vi "Auton_S1_Left_Scale_2Cube.vi"   [LabVIEW 2017]
uses:
  <vilib>/Rock Robotics/WPI/Utilities/WPI_GetSetVariantRefNum.vi
  Robot Global Data.vi
  <vilib>/Rock Robotics/WPI/RobotDrive/WPI_RobotDriveArcadeDrive_Standard(NoSaturation).vi
types:
  T1 = typedef "WPI_RobotDriveDevRef.ctl" = cluster{"DevStatus":errorcluster, "Motors[]":T2[], "Square Inputs":bool, "Max Output":dbl}
  T2 = typedef "WPI_MotorControlDeviceRef.ctl" = cluster{"DeviceStatus":errorcluster, "Type":T3, "PWM":cluster{"PWM Channel":T4, "DeadBand":T5}, "CAN":cluster{"Device Number":u8, "SetOutput VI Ref":variant, "GetOutput VI Ref":variant, "Enable VI Ref":variant, "Disable VI Ref":variant, "Data":variant}, "Invert":bool, "DIO PWM":cluster{"PWM \"Enable\" Channel":T4, "DIOChannel":T6, "PWM Rate":dbl}}
  T3 = typedef "WPI_MotorControlType.ctl" = enum16{"PWM", "CAN", "DIO PWM"}
  T4 = typedef "FPGA_DIOPWMChannel.ctl" = enum8{"PWM 0", "PWM 1", "PWM 2", "PWM 3", "PWM 4", "PWM 5", "PWM 6", "PWM 7", "PWM 8", "PWM 9", "PWM MXP 0", "PWM MXP 1", "PWM MXP 2", "PWM MXP 3", "PWM MXP 4", "PWM MXP 5", "PWM MXP 6", "PWM MXP 7", "PWM MXP 8", "PWM MXP 9", "Invalid"}
  T5 = typedef "WPI_PWMDeadband.ctl" = cluster{"Name":string, "maxPositivePwm":i32, "minPositivePwm":i32, "centerPwm":i32, "maxNegativePwm":i32, "minNegativePwm":i32, "angularRange":u16}
  T6 = typedef "FPGA_DIOChannel.ctl" = enum8{"DIO 0", "DIO 1", "DIO 2", "DIO 3", "DIO 4", "DIO 5", "DIO 6", "DIO 7", "DIO 8", "DIO 9", "DIO MXP 0", "DIO MXP 1", "DIO MXP 2", "DIO MXP 3", "DIO MXP 4", "DIO MXP 5", "DIO MXP 6", "DIO MXP 7", "DIO MXP 8", "DIO MXP 9", "DIO MXP 10", "DIO MXP 11", "DIO MXP 12", "DIO MXP 13", "DIO MXP 14", "DIO MXP 15", "SPI Port CS1", "SPI Port CS2", "SPI Port CS3", "SPI Port MISO", "SPI Port MOSI", "Invalid"}
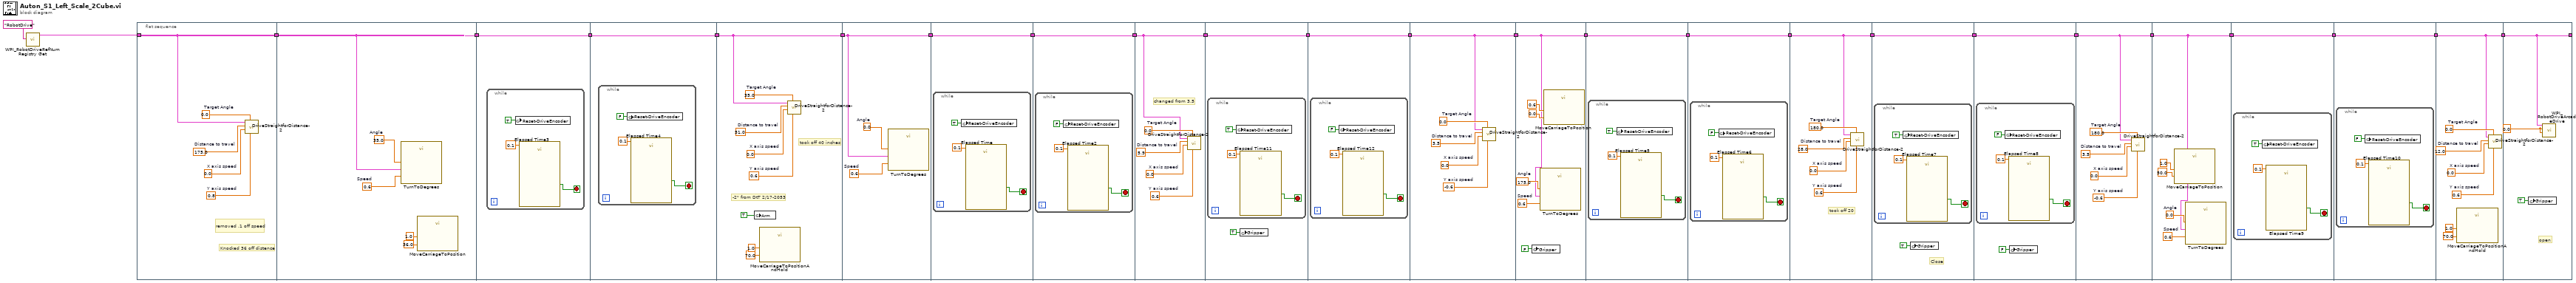
[diagram p0: block diagram]
diagram:
  n1 = call <vilib>:"WPI_RobotDriveRefNum Registry Get.vi"("refnum name"="RobotDrive") -> ("RobotDriveDevRef"=w22:T1)  [unwired: 9 in, 1 out]
  n2 = flat-sequence {
    tunnel: [w30] -> w1
    tunnel: w22 -> [w30]
    tunnel: [w34] -> w25
    tunnel: w1 -> [w34]
    tunnel: w25 -> [w36]
    tunnel: [w36] -> w24
    tunnel: [w40] -> w21
    tunnel: w24 -> [w40]
    tunnel: w21 -> [w47]
    tunnel: [w47] -> w7
    tunnel: w7 -> [w52]
    tunnel: [w52] -> w6
    tunnel: w6 -> [w55]
    tunnel: [w55] -> w20
    tunnel: w20 -> [w59]
    tunnel: [w59] -> w19
    tunnel: w19 -> [w63]
    tunnel: [w63] -> w5
    tunnel: w5 -> [w69]
    tunnel: [w69] -> w3
    tunnel: w3 -> [w73]
    tunnel: [w73] -> w2
    tunnel: w2 -> [w77]
    tunnel: [w77] -> w4
    tunnel: w4 -> [w83]
    tunnel: [w83] -> w18
    tunnel: w18 -> [w88]
    tunnel: [w88] -> w17
    tunnel: w17 -> [w92]
    tunnel: [w92] -> w16
    tunnel: w16 -> [w96]
    tunnel: [w96] -> w15
    tunnel: w15 -> [w102]
    tunnel: [w102] -> w14
    tunnel: w14 -> [w107]
    tunnel: [w107] -> w13
    tunnel: w13 -> [w111]
    tunnel: [w111] -> w12
    tunnel: w12 -> [w118]
    tunnel: [w118] -> w11
    tunnel: w11 -> [w121]
    tunnel: [w121] -> w10
    tunnel: w10 -> [w125]
    tunnel: [w125] -> w9
    tunnel: w9 -> [w131]
    tunnel: [w131] -> w8
    tunnel: [w137] -> _
    tunnel: w8 -> [w137]
    frame #0 {
      w26 = 0.0  # Target Angle
      w27 = 0.8  # Y axis speed
      w28 = 0.0  # X axis speed
      w29 = 175.0  # Distance to travel
      # "removed .1 off speed"
      # "Knocked 36 off distence"
      n3 = call "DriveStraightforDistance-2.vi"("Y axis speed"=w27, "Target Angle"=w26, "X axis speed"=w28, "Distance to travel"=w29, "RobotDriveDevRef"=w30) -> ()  [unwired: 7 in]
    }
    frame #1 {
      w33 = 35.0  # Angle
      w35 = 0.6  # Speed
      n4 = call "TurnToDegrees.vi"("Speed"=w35, "RobotDriveDevRef"=w34, "Angle"=w33) -> ()  [unwired: 9 in]
      n5 = call "MoveCarriageToPosition.vi"("Lift Speed"=1.0, "Target Height"=36.0) -> ()  [unwired: 10 in]
    }
    frame #2 {
      n6 = while {
        stop <- w39 stop-if-true
        n7 = global write "Robot Global Data.vi" "Reset-DriveEncoder"(TRUE ("Reset-DriveEncoder")) -> ()
        n8 = call "Elapsed Time3"("Time Target (s)"=0.1) -> ("Time has Elapsed"=w39:bool)  [unwired: 11 in, 7 out]
      }
    }
    frame #3 {
      n9 = while {
        stop <- w43 stop-if-true
        n10 = global write "Robot Global Data.vi" "Reset-DriveEncoder"(FALSE ("Reset-DriveEncoder")) -> ()
        n11 = call "Elapsed Time4"("Time Target (s)"=0.1) -> ("Time has Elapsed"=w43:bool)  [unwired: 11 in, 7 out]
      }
    }
    frame #4 {
      w48 = 35.0  # Target Angle
      w49 = 0.6  # Y axis speed
      w50 = 0.0  # X axis speed
      w51 = 51.0  # Distance to travel
      # "took off 40 inches"
      # "-2\" from DtT 2/17-2053"
      n12 = global write "Robot Global Data.vi" "Arm"(TRUE ("Gripper")) -> ()
      n13 = call "MoveCarriageToPositionAndHold.vi"("Lift Speed"=1.0, "Target Height"=70.0) -> ()  [unwired: 10 in]
      n14 = call "DriveStraightforDistance-2.vi"("Y axis speed"=w49, "Target Angle"=w48, "X axis speed"=w50, "Distance to travel"=w51, "RobotDriveDevRef"=w47) -> ()  [unwired: 7 in]
    }
    frame #5 {
      w53 = 0.0  # Angle
      w54 = 0.6  # Speed
      n15 = call "TurnToDegrees.vi"("Speed"=w54, "RobotDriveDevRef"=w52, "Angle"=w53) -> ()  [unwired: 9 in]
    }
    frame #6 {
      n16 = while {
        stop <- w58 stop-if-true
        n17 = global write "Robot Global Data.vi" "Reset-DriveEncoder"(TRUE ("Reset-DriveEncoder")) -> ()
        n18 = call "Elapsed Time"("Time Target (s)"=0.1) -> ("Time has Elapsed"=w58:bool)  [unwired: 11 in, 7 out]
      }
    }
    frame #7 {
      n19 = while {
        stop <- w62 stop-if-true
        n20 = global write "Robot Global Data.vi" "Reset-DriveEncoder"(FALSE ("Reset-DriveEncoder")) -> ()
        n21 = call "Elapsed Time2"("Time Target (s)"=0.1) -> ("Time has Elapsed"=w62:bool)  [unwired: 11 in, 7 out]
      }
    }
    frame #8 {
      w64 = 0.0  # Target Angle
      w65 = 0.6  # Y axis speed
      w66 = 0.0  # X axis speed
      w67 = 5.9  # Distance to travel
      # "changed from 3.5"
      n22 = call "DriveStraightforDistance-2.vi"("Y axis speed"=w65, "Target Angle"=w64, "X axis speed"=w66, "Distance to travel"=w67, "RobotDriveDevRef"=w63) -> ()  [unwired: 7 in]
    }
    frame #9 {
      n23 = while {
        stop <- w72 stop-if-true
        n24 = global write "Robot Global Data.vi" "Reset-DriveEncoder"(TRUE ("Reset-DriveEncoder")) -> ()
        n25 = call "Elapsed Time11"("Time Target (s)"=0.1) -> ("Time has Elapsed"=w72:bool)  [unwired: 11 in, 7 out]
      }
      n26 = global write "Robot Global Data.vi" "Gripper"(TRUE ("Gripper")) -> ()
    }
    frame #10 {
      n27 = while {
        stop <- w76 stop-if-true
        n28 = global write "Robot Global Data.vi" "Reset-DriveEncoder"(FALSE ("Reset-DriveEncoder")) -> ()
        n29 = call "Elapsed Time12"("Time Target (s)"=0.1) -> ("Time has Elapsed"=w76:bool)  [unwired: 11 in, 7 out]
      }
    }
    frame #11 {
      w78 = 0.0  # Target Angle
      w79 = -0.6  # Y axis speed
      w80 = 0.0  # X axis speed
      w81 = 3.5  # Distance to travel
      n30 = call "DriveStraightforDistance-2.vi"("Y axis speed"=w79, "Target Angle"=w78, "X axis speed"=w80, "Distance to travel"=w81, "RobotDriveDevRef"=w77) -> ()  [unwired: 7 in]
    }
    frame #12 {
      w84 = 175.0  # Angle
      w85 = 0.6  # Speed
      n31 = global write "Robot Global Data.vi" "Gripper"(FALSE ("Gripper")) -> ()
      n32 = call "TurnToDegrees.vi"("Speed"=w85, "RobotDriveDevRef"=w83, "Angle"=w84) -> ()  [unwired: 9 in]
      n33 = call "MoveCarriageToPosition.vi"("Lift Speed"=0.6, "Target Height"=0.0) -> ()  [unwired: 10 in]
    }
    frame #13 {
      n34 = while {
        stop <- w91 stop-if-true
        n35 = global write "Robot Global Data.vi" "Reset-DriveEncoder"(TRUE ("Reset-DriveEncoder")) -> ()
        n36 = call "Elapsed Time5"("Time Target (s)"=0.1) -> ("Time has Elapsed"=w91:bool)  [unwired: 11 in, 7 out]
      }
    }
    frame #14 {
      n37 = while {
        stop <- w95 stop-if-true
        n38 = global write "Robot Global Data.vi" "Reset-DriveEncoder"(FALSE ("Reset-DriveEncoder")) -> ()
        n39 = call "Elapsed Time6"("Time Target (s)"=0.1) -> ("Time has Elapsed"=w95:bool)  [unwired: 11 in, 7 out]
      }
    }
    frame #15 {
      w97 = 180.0  # Target Angle
      w98 = 0.6  # Y axis speed
      w99 = 0.0  # X axis speed
      w100 = 28.0  # Distance to travel
      # "took off 20"
      n40 = call "DriveStraightforDistance-2.vi"("Y axis speed"=w98, "Target Angle"=w97, "X axis speed"=w99, "Distance to travel"=w100, "RobotDriveDevRef"=w96) -> ()  [unwired: 7 in]
    }
    frame #16 {
      # "Close"
      n41 = while {
        stop <- w105 stop-if-true
        n42 = global write "Robot Global Data.vi" "Reset-DriveEncoder"(TRUE ("Reset-DriveEncoder")) -> ()
        n43 = call "Elapsed Time7"("Time Target (s)"=0.1) -> ("Time has Elapsed"=w105:bool)  [unwired: 11 in, 7 out]
      }
      n44 = global write "Robot Global Data.vi" "Gripper"(TRUE ("Gripper")) -> ()
    }
    frame #17 {
      n45 = while {
        stop <- w110 stop-if-true
        n46 = global write "Robot Global Data.vi" "Reset-DriveEncoder"(FALSE ("Reset-DriveEncoder")) -> ()
        n47 = call "Elapsed Time8"("Time Target (s)"=0.1) -> ("Time has Elapsed"=w110:bool)  [unwired: 11 in, 7 out]
      }
      n48 = global write "Robot Global Data.vi" "Gripper"(FALSE ("Gripper")) -> ()
    }
    frame #18 {
      w112 = 180.0  # Target Angle
      w113 = -0.6  # Y axis speed
      w114 = 0.0  # X axis speed
      w115 = 3.5  # Distance to travel
      n49 = call "DriveStraightforDistance-2.vi"("Y axis speed"=w113, "Target Angle"=w112, "X axis speed"=w114, "Distance to travel"=w115, "RobotDriveDevRef"=w111) -> ()  [unwired: 7 in]
    }
    frame #19 {
      w119 = 0.0  # Angle
      w120 = 0.6  # Speed
      n50 = call "MoveCarriageToPosition.vi"("Lift Speed"=1.0, "Target Height"=50.0) -> ()  [unwired: 10 in]
      n51 = call "TurnToDegrees.vi"("Speed"=w120, "RobotDriveDevRef"=w118, "Angle"=w119) -> ()  [unwired: 9 in]
    }
    frame #20 {
      n52 = while {
        stop <- w124 stop-if-true
        n53 = global write "Robot Global Data.vi" "Reset-DriveEncoder"(TRUE ("Reset-DriveEncoder")) -> ()
        n54 = call "Elapsed Time9"("Time Target (s)"=0.1) -> ("Time has Elapsed"=w124:bool)  [unwired: 11 in, 7 out]
      }
    }
    frame #21 {
      n55 = while {
        stop <- w128 stop-if-true
        n56 = global write "Robot Global Data.vi" "Reset-DriveEncoder"(FALSE ("Reset-DriveEncoder")) -> ()
        n57 = call "Elapsed Time10"("Time Target (s)"=0.1) -> ("Time has Elapsed"=w128:bool)  [unwired: 11 in, 7 out]
      }
    }
    frame #22 {
      w132 = 0.0  # Target Angle
      w133 = 0.6  # Y axis speed
      w134 = 0.0  # X axis speed
      w135 = 12.0  # Distance to travel
      n58 = call "MoveCarriageToPositionAndHold.vi"("Lift Speed"=1.0, "Target Height"=70.0) -> ()  [unwired: 10 in]
      n59 = call "DriveStraightforDistance-2.vi"("Y axis speed"=w133, "Target Angle"=w132, "X axis speed"=w134, "Distance to travel"=w135, "RobotDriveDevRef"=w131) -> ()  [unwired: 7 in]
    }
    frame #23 {
      w138 = 0.0 ("X axis value")
      # "open"
      n60 = global write "Robot Global Data.vi" "Gripper"(TRUE ("Gripper")) -> ()
      n61 = call-poly <vilib>:"WPI_RobotDriveArcadeDrive.vi"("Y axis value"=w138, "X axis value"=w138, "RobotDriveDevRef"=w137) -> ()  [unwired: 6 in, 3 out]
    }
  }
